vi "Miniquads.constructor.vi"(0 "name":string, 2 "data in":string, 5 "error in (no error)":errorcluster) -> (14 "i ref out":refnum<vi>, 16 "data out":string, 19 "error out":errorcluster)   [LabVIEW 2014, in "Miniquads.lvlib"]
doc: "This is the constructor of a class.\n\nLicense Agreement for this software:\n\nCopyright (C) 2011 Christopher Borgmann\nMax-Planck-Institut für Kernphysik\nSaupfercheckweg 1\n69117 Heidelberg\nGermany\n\nThis program is free software: you can redistribute it and/or modify it under the terms of the GNU General Public License as published by the Free Software Foundation, either version 3 of the License, or (at your option) any later version.\n\nThis program is distributed in the hope that it will be useful, but WITHOUT ANY WARRANTY; without even the implied warranty of MERCHANTABILITY or FITNESS FOR A PARTICULAR PURPOSE. See the GNU General Public License for more details.\n\nYou should have received a copy of the GNU General Public License along with this program. If not, see <http://www.gnu.org/licenses/>.\n\nFor all questions and ideas contact: christopher.borgmann@cern.ch."
uses:
  Miniquads.lvlib
  Miniquads.i attribute.ctl
  Miniquads.voltages.ctl
  CS_Core/CSApplicationBaseClasses/DeviceBase/DeviceBase.myEventNames.ctl
  CS_Core/CSApplicationBaseClasses/DeviceBase/DeviceBase.lvlib
  CS_Core/CSSystem/CSSystemLib/CSSystemLib.lvlib
panel:
  in  "attributeType":T1
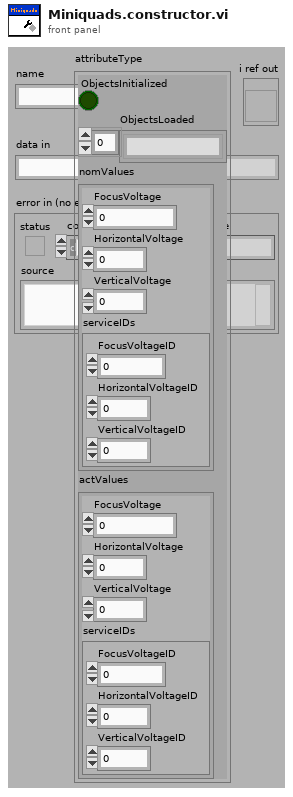
[diagram p1: front panel]
types:
  T1 = typedef "Miniquads.lvlib/Miniquads.i attribute.ctl" = cluster{"ObjectsInitialized":bool, "ObjectsLoaded":string[], "nomValues":T2, "actValues":T2}
  T2 = typedef "Miniquads.lvlib/Miniquads.voltages.ctl" = cluster{"FocusVoltage":dbl, "HorizontalVoltage":dbl, "VerticalVoltage":dbl, "serviceIDs":cluster{"FocusVoltageID":i32, "HorizontalVoltageID":i32, "VerticalVoltageID":i32}}
  T3 = enum16{"SetAttribute", "GetAttribute", "CreateAttribute", "DestroyAttribute", "DestroyAllAtributes"}
  T4 = typedef "DeviceBase.lvlib/DeviceBase.myEventNames.ctl" = enum16{"lvmsg://Initialize", "lvmsg://Close", "lvmsg://Configure", "lvmsg://Reset", "lvmsg://IDQuery"}
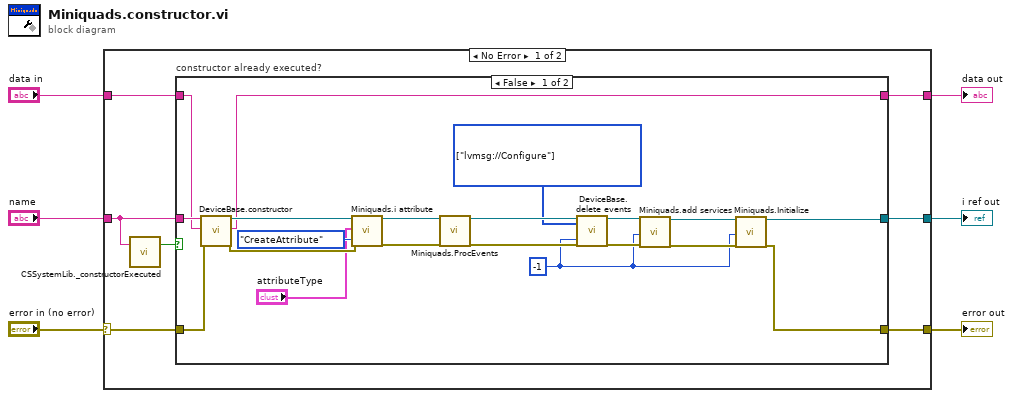
[diagram p0: block diagram]
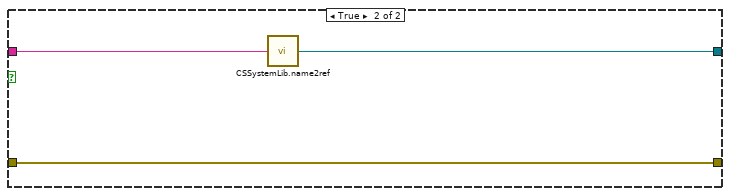
[diagram p2: hidden frame]
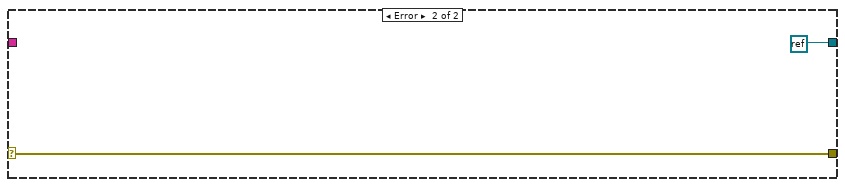
[diagram p3: hidden frame]
diagram:
  n1 = case shown="No Error" "error in (no error)" {
    selector: "error in (no error)" -> [w11 w37]
    tunnel: "name" -> [w10 _]
    tunnel: [w13 refnum<k0> refnum ("Not a Refnum Constant")] -> w5
    tunnel: [w12 w37] -> w4
    tunnel: "data in" -> [w8 _]
    tunnel: [w7 _] -> w1
    frame No Error {
      n2 = call "CSSystemLib._constructorExecuted.vi"("name"=w10) -> ("constructor executed?"=w9:bool)  [unwired: 18 in]
      n3 = case "constructor already executed?" shown="False" w9 {
        tunnel: w10 -> [w30 w36]
        tunnel: [w17 w35] -> w13
        tunnel: [w16 w34] -> w12
        tunnel: w11 -> [w27 w34]
        tunnel: w8 -> [w26 _]
        tunnel: [w22 _] -> w7
        frame False {
          w23 = T4[] [enum."lvmsg://Configure"] items=["lvmsg://Initialize", "lvmsg://Close", "lvmsg://Configure", "lvmsg://Reset", "lvmsg://IDQuery"] ("events")
          w14 = -1 ("ms timeout (10000)")
          n4 = call "DeviceBase.constructor.vi"("name"=w30, "data in"=w26, "error in (no error)"=w27) -> ("i ref out"=w33:refnum<vi>, "data out"=w22:string, "error out"=w32:errorcluster)  [unwired: 14 in]
          n5 = call "Miniquads.i attribute.vi"("VI Refnum"=w33, "CLASS.i attribute"="attributeType", "Action"=T3."CreateAttribute", "error in (no error)"=w32) -> ("VI Refnum out"=w29:refnum<vi>, "error out"=w28:errorcluster)  [unwired: 13 in, 1 out]
          n6 = call "Miniquads.ProcEvents.vi"("i ref in"=w29, "error in (no error)"=w28) -> ("i ref out"=w25:refnum<vi>, "error out"=w24:errorcluster)  [unwired: 16 in]
          n7 = call "DeviceBase.delete events.vi"("i ref in"=w25, "events"=w23, "ms timeout (10000)"=w14, "error in (no error)"=w24) -> ("i ref out"=w19:refnum<vi>, "error out"=w20:errorcluster)  [unwired: 13 in, 1 out]
          n8 = call "Miniquads.add services.vi"("i ref in"=w19, "ms timeout (10000)"=w14, "error in (no error)"=w20) -> ("i ref out"=w18:refnum<vi>, "error out"=w15:errorcluster)  [unwired: 14 in, 1 out]
          n9 = call "Miniquads.Initialize.vi"("i ref in"=w18, "ms timeout (10000)"=w14, "error in (no error)"=w15) -> ("i ref out"=w17:refnum<vi>, "error out"=w16:errorcluster)  [unwired: 13 in, 2 out]
        }
        frame True {
          n10 = call "CSSystemLib.name2ref.vi"("name"=w36) -> ("obj refnum"=w35:refnum<vi>)
        }
      }
    }
    frame Error {
    }
  }
  "i ref out" <- w5
  "error out" <- w4
  "data out" <- w1
